vi "stub_Get Cells.vi"   [LabVIEW 2013]
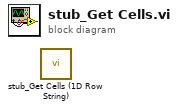
[diagram p0: block diagram]
diagram:
  n1 = call "stub_Get Cells (1D Row String).vi"() -> ()  [unwired: 9 in, 3 out]
